vi "Realsense Cam Create.vi"(7 "Connect? (T)":bool=TRUE, 8 "error in (no error)":errorcluster, 9 "Sensor Index (0)":i32, 10 "Device Index (0)":i32, 11 "Realsense Cam in":refnum<class "Realsense Cam.lvclass">) -> (0 "error out":errorcluster, 1 "init error":string="No Error\rNo Error\rNo Error\rNo Error\rNo Error\rNo Error\rNo Error\rNo Error\rNo Error\rNo Error\rNo Error", 2 "Found?":bool, 3 "Realsense Cam out":refnum<class "Realsense Cam.lvclass">)   [LabVIEW 2018, in "Realsense Cam.lvclass"]
uses:
  Realsense Cam.lvclass
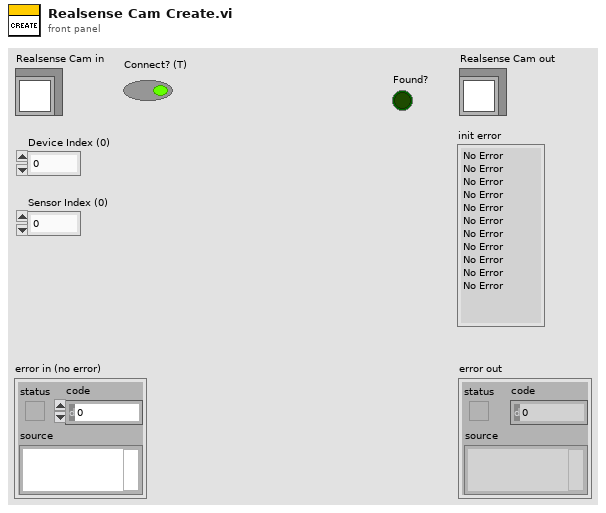
[diagram p1: front panel]
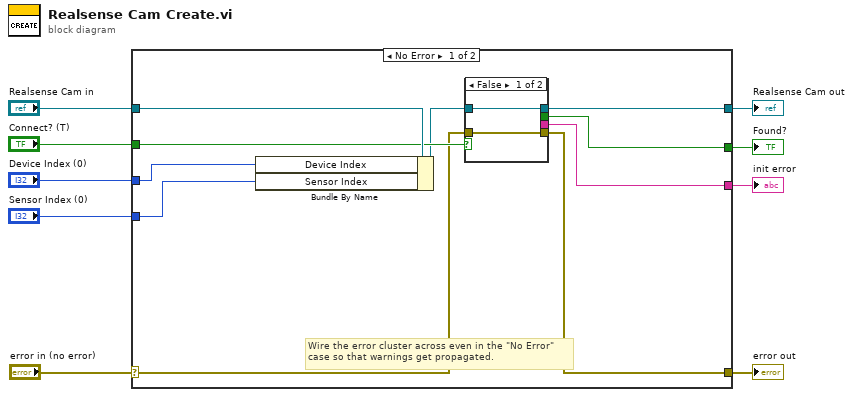
[diagram p0: block diagram]
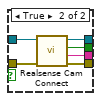
[diagram p2: hidden frame]
diagram:
  n1 = case shown="No Error" "error in (no error)" {
    selector: "error in (no error)" -> [w11 w29]
    tunnel: [w10 w29] -> w8
    tunnel: [w14 w28] -> w6
    tunnel: "Realsense Cam in" -> [w19 w28]
    tunnel: "Connect? (T)" -> [w16 _]
    tunnel: "Device Index (0)" -> [w18 _]
    tunnel: "Sensor Index (0)" -> [w17 _]
    tunnel: [w13 _] -> w2
    tunnel: [w12 _] -> w1
    frame No Error {
      # "Wire the error cluster across even in the \"No Error\"\ncase so that warnings get propagated."
      n2 = Bundle By Name(cluster=w19, "Device Index"=w18, "Sensor Index"=w17) -> (w15:refnum<class "Realsense Cam.lvclass">)
      n3 = case shown="False" w16 {
        tunnel: w15 -> [w21 w27]
        tunnel: [w21 w26] -> w14
        tunnel: [_ w25] -> w13
        tunnel: [_ w24] -> w12
        tunnel: w11 -> [w20 w23]
        tunnel: [w20 w22] -> w10
        frame False {
        }
        frame True {
          n4 = call-dynamic "Realsense Cam Connect.vi"("error in (no error)"=w23, "Realsense Cam in"=w27) -> ("error out"=w22:errorcluster, "init error"=w24:string, "Found?"=w25:bool, "Realsense Cam out"=w26:refnum<class "Realsense Cam.lvclass">)  [unwired: 6 in]
        }
      }
    }
    frame Error {
    }
  }
  "error out" <- w8
  "Realsense Cam out" <- w6
  "Found?" <- w2
  "init error" <- w1
